vi "test_libssh2_userauth_list.vi"() -> ()   [LabVIEW 2017, in "integration_tests.lvlib"]
uses:
  integration_tests.lvlib
  libssh2/libssh2_session_handshake_tcp.vi
  libssh2/libssh2_init_default.vi
  libssh2/libssh2_session_init_ex.vi
  <vilib>/Utility/tcp.llb/TCP Get Raw Net Object.vi
  libssh2/libssh2_session_handshake_socket.vi
  libssh2/libssh2.lvlib
  support/support.lvlib
  <vilib>/PNR/Transparent Assertions/Transparent Assertions/Transparent Assertions.lvlib
panel:
  out "error out":errorcluster
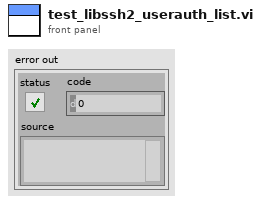
[diagram p1: front panel]
types:
  T1 = typedef "libssh2.lvlib/Session Refnum.ctl" = refnum<k1>
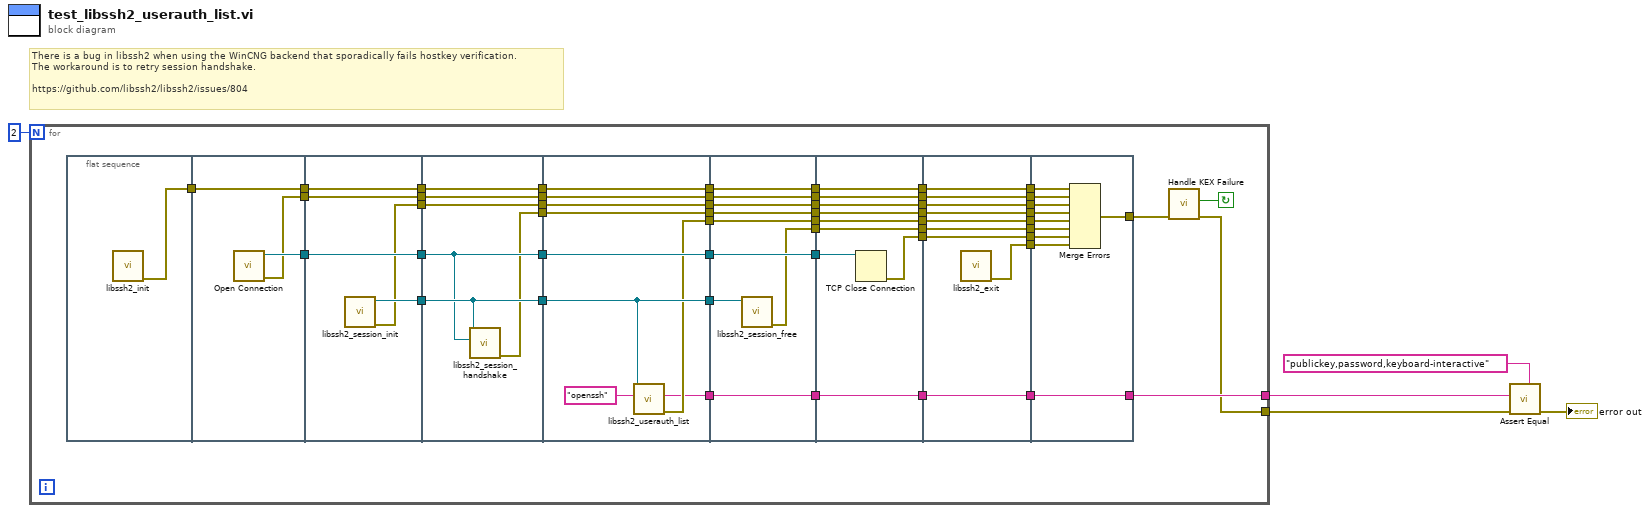
[diagram p0: block diagram]
diagram:
  # "There is a bug in libssh2 when using the WinCNG backend that sporadically fails hostkey verification.\nThe workaround is to retry session handshake.\n\nhttps://github.com/libssh2/libssh2/issues/804"
  n1 = for {
    N: 2 -> [_]
    tunnel: [w9] -> w3
    tunnel: [w6] -> w2
    stop <- w7 continue-if-true
    n2 = flat-sequence {
      tunnel: [w58] -> w57
      tunnel: [w61] -> w56
      tunnel: w57 -> [w60]
      tunnel: [w60] -> w55
      tunnel: [w59] -> w54
      tunnel: w56 -> [w66]
      tunnel: [w66] -> w53
      tunnel: w55 -> [w65]
      tunnel: [w65] -> w52
      tunnel: w54 -> [w64]
      tunnel: [w64] -> w51
      tunnel: [w63] -> w50
      tunnel: [w62] -> w49
      tunnel: w53 -> [w68]
      tunnel: [w68] -> w48
      tunnel: w52 -> [w72]
      tunnel: [w72] -> w47
      tunnel: w51 -> [w71]
      tunnel: [w71] -> w46
      tunnel: [w70] -> w45
      tunnel: w50 -> [w70]
      tunnel: w49 -> [w69]
      tunnel: [w69] -> w44
      tunnel: [w67] -> w43
      tunnel: w48 -> [w81]
      tunnel: [w81] -> w42
      tunnel: w47 -> [w80]
      tunnel: [w80] -> w41
      tunnel: w46 -> [w79]
      tunnel: [w79] -> w40
      tunnel: w45 -> [w76]
      tunnel: w44 -> [w78]
      tunnel: [w78] -> w39
      tunnel: w43 -> [w77]
      tunnel: [w77] -> w38
      tunnel: [w75] -> w37
      tunnel: [w76] -> w35
      tunnel: [w73] -> w36
      tunnel: w42 -> [w90]
      tunnel: [w90] -> w34
      tunnel: w41 -> [w89]
      tunnel: [w89] -> w33
      tunnel: w40 -> [w88]
      tunnel: [w88] -> w32
      tunnel: w39 -> [w87]
      tunnel: [w87] -> w31
      tunnel: w38 -> [w86]
      tunnel: [w86] -> w30
      tunnel: w37 -> [w85]
      tunnel: [w85] -> w29
      tunnel: [w84] -> w28
      tunnel: [w83] -> w27
      tunnel: w36 -> [w83]
      tunnel: w35 -> [w82]
      tunnel: w34 -> [w99]
      tunnel: w33 -> [w98]
      tunnel: [w98] -> w26
      tunnel: w32 -> [w97]
      tunnel: [w97] -> w25
      tunnel: [w96] -> w24
      tunnel: w31 -> [w95]
      tunnel: [w95] -> w23
      tunnel: w30 -> [w94]
      tunnel: [w94] -> w22
      tunnel: w29 -> [w93]
      tunnel: [w93] -> w21
      tunnel: [w92] -> w20
      tunnel: w28 -> [w92]
      tunnel: [w91] -> w19
      tunnel: w27 -> [w91]
      tunnel: w26 -> [w108]
      tunnel: [w108] -> w18
      tunnel: w25 -> [w107]
      tunnel: [w107] -> w17
      tunnel: w24 -> [w106]
      tunnel: [w106] -> w16
      tunnel: [w105] -> w15
      tunnel: w23 -> [w104]
      tunnel: [w104] -> w14
      tunnel: w22 -> [w103]
      tunnel: [w103] -> w13
      tunnel: w21 -> [w102]
      tunnel: [w102] -> w12
      tunnel: [w101] -> w11
      tunnel: w20 -> [w101]
      tunnel: [w100] -> w10
      tunnel: w19 -> [w100]
      tunnel: w18 -> [w118]
      tunnel: w17 -> [w117]
      tunnel: w16 -> [w116]
      tunnel: w15 -> [w115]
      tunnel: w14 -> [w114]
      tunnel: w13 -> [w113]
      tunnel: w12 -> [w112]
      tunnel: w11 -> [w111]
      tunnel: w10 -> [w110]
      tunnel: [w110] -> w9
      tunnel: [w109] -> w8
      frame #0 {
        n3 = call-poly "libssh2_init.vi"() -> ("error out"=w58:errorcluster)  [unwired: 11 in]
      }
      frame #1 {
        n4 = call "Open Connection.vi"() -> ("error out"=w59:errorcluster, "connection ID"=w61:refnum<k5>)  [unwired: 10 in]
      }
      frame #2 {
        n5 = call "libssh2_session_init.vi"() -> ("error out"=w62:errorcluster, "session"=w63:T1)  [unwired: 10 in]
      }
      frame #3 {
        n6 = call-poly "libssh2_session_handshake.vi"("tcp connection"=w68, "session"=w70) -> ("error out"=w67:errorcluster)  [unwired: 9 in]
      }
      frame #4 {
        n7 = call "libssh2_userauth_list.vi"("username"="openssh", "session"=w76) -> ("error out"=w75:errorcluster, "supported authentication schemes"=w73:string)  [unwired: 8 in]
      }
      frame #5 {
        n8 = call "libssh2_session_free.vi"("session"=w82) -> ("error out"=w84:errorcluster)  [unwired: 10 in]
      }
      frame #6 {
        n9 = TCP Close Connection(connection ID=w99) -> (error out=w96:errorcluster)  [unwired: 2 in, 1 out]
      }
      frame #7 {
        n10 = call "libssh2_exit.vi"() -> ("error out"=w105:errorcluster)  [unwired: 11 in]
      }
      frame #8 {
        n11 = Merge Errors(w118, w117, w114, w113, w112, w111, w116, w115) -> (w109:errorcluster)
      }
    }
    n12 = call "Handle KEX Failure.vi"("error in (no error)"=w8) -> ("error out"=w6:errorcluster, "KEX Failure"=w7:bool)  [unwired: 9 in]
  }
  n13 = call <vilib>:"Assert Equal.vi"("Expected"="publickey,password,keyboard-interactive" ("supported authentication schemes"), "error in (no error)"=w2, "Actual"=w3) -> ("error out"=→"error out":errorcluster)  [unwired: 8 in]
